vi "TCP Check - Client.vi"(0 "remote port or service name":u16, 1 "address":string="127.0.0.1", 3 "error in (no error)":errorcluster) -> (8 "Connection Established":bool, 9 "Message from Server":string, 10 "error out":errorcluster)   [LabVIEW 2020]
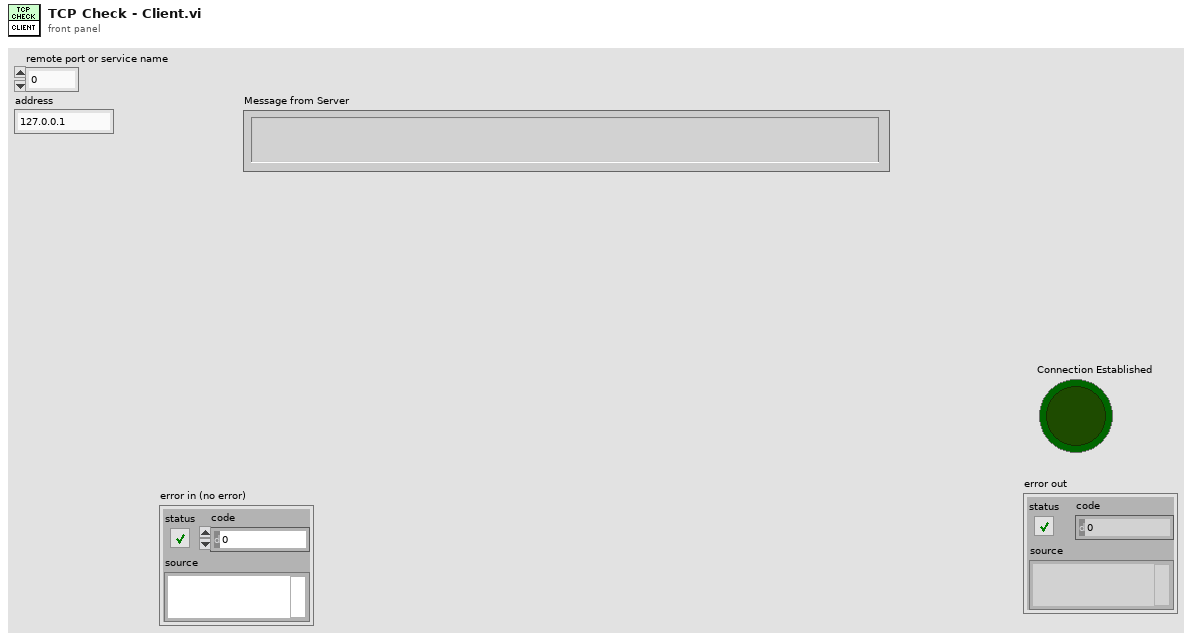
[diagram p1: front panel]
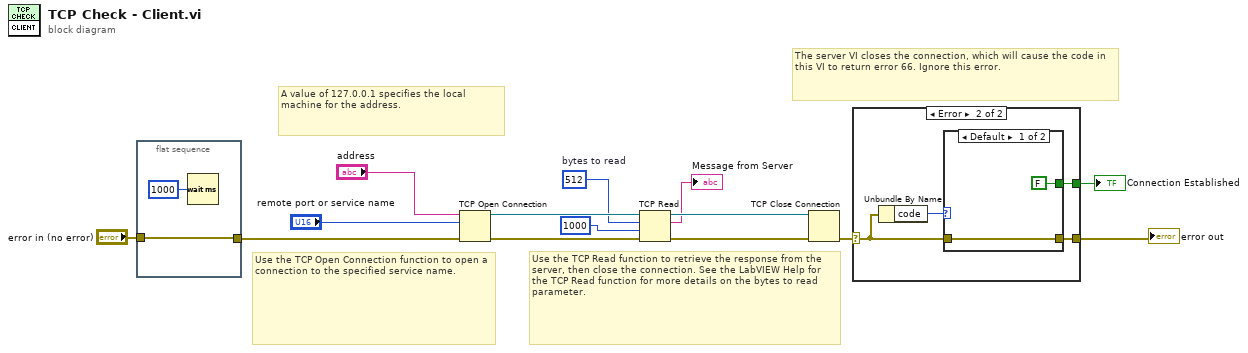
[diagram p0: block diagram]
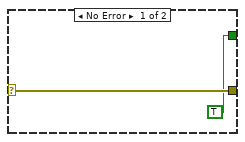
[diagram p2: hidden frame]
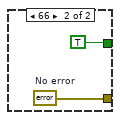
[diagram p3: hidden frame]
diagram:
  w8 = 512  # bytes to read
  # "The server VI closes the connection, which will cause the code in this VI to return error 66. Ignore this error."
  # "A value of 127.0.0.1 specifies the local machine for the address."
  # "Use the TCP Open Connection function to open a connection to the specified service name."
  # "Use the TCP Read function to retrieve the response from the server, then close the connection. See the LabVIEW Help for the TCP Read function for more details on the bytes to read parameter."
  n1 = flat-sequence {
    tunnel: "error in (no error)" -> [w15]
    tunnel: [w15] -> w3
    frame #0 {
      n2 = Wait (ms)(milliseconds to wait=u32 1000) -> ()  [unwired: 1 out]
    }
  }
  n3 = TCP Open Connection(address="address", remote port or service name="remote port or service name", error in (no error)=w3) -> (connection ID=w13:refnum<k5>, error out=w14:errorcluster)  [unwired: 2 in]
  n4 = TCP Read(connection ID=w13, bytes to read=w8, error in (no error)=w14, 9:1000 ("timeout ms (60000)")) -> (connection ID out=w12:refnum<k5>, data out=→"Message from Server":string, error out=w11:errorcluster)  [unwired: 1 in]
  n5 = TCP Close Connection(connection ID=w12, error in (no error)=w11) -> (error out=w7:errorcluster)  [unwired: 1 in, 1 out]
  n6 = case shown="Error" w7 {
    selector: w7 -> [w18 w21]
    tunnel: [w18 w20] -> w6
    tunnel: [TRUE w19] -> w5
    frame No Error {
    }
    frame Error {
      n7 = Unbundle By Name(w21) -> ("code"=w22:i32)
      n8 = case shown="Default" w22 {
        tunnel: w21 -> [w24 _]
        tunnel: [w24 w26] -> w20
        tunnel: [FALSE TRUE] -> w19
        frame Default {
        }
        frame 66 {
          w26 = errorcluster {"status"=FALSE, "code"=0, "source"=""}  # No error
        }
      }
    }
  }
  "error out" <- w6
  "Connection Established" <- w5
